vi "zerolevel.vi"(7 "Zerolevel on?":bool, 8 "Power in":dbl, 9 "rho-":dbl[](array[numeric]), 10 "rho0":dbl[](array[numeric]), 11 "rho+":dbl[](array[numeric])) -> (1 "rho- out":dbl[](array[numeric]), 2 "rho0 out":dbl[](array[numeric]), 3 "rho+ out":dbl[](array[numeric]))   [LabVIEW 2018]
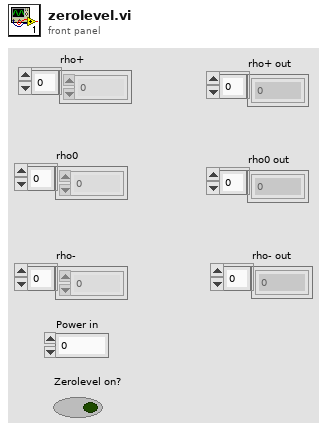
[diagram p1: front panel]
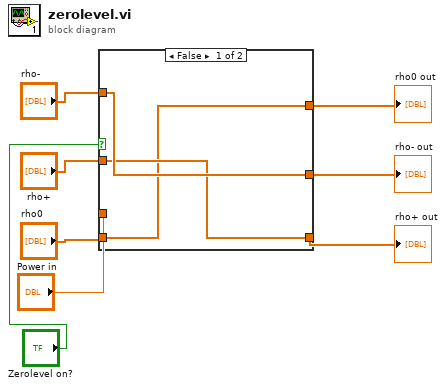
[diagram p0: block diagram]
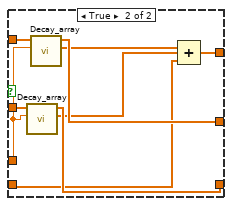
[diagram p2: hidden frame]
diagram:
  n1 = case shown="False" "Zerolevel on?" {
    tunnel: "rho-" -> [w11 w20]
    tunnel: [w11 w19] -> w7
    tunnel: "rho+" -> [w10 w18]
    tunnel: "Power in" -> [_ w17]
    tunnel: [w10 w16] -> w4
    tunnel: "rho0" -> [w9 w13]
    tunnel: [w9 w12] -> w2
    frame False {
    }
    frame True {
      n2 = call "Decay_array.vi"("Power in"=w17, "Array in"=w18) -> ("Change out"=w14:dbl[], "Array out"=w16:dbl[])  [unwired: 8 in]
      n3 = call "Decay_array.vi"("Power in"=w17, "Array in"=w20) -> ("Change out"=w15:dbl[], "Array out"=w19:dbl[])  [unwired: 8 in]
      n4 = Compound Arithmetic op=ADD(w15, w14, w13) -> (w12:dbl[])
    }
  }
  "rho+ out" <- w4
  "rho0 out" <- w2
  "rho- out" <- w7
